vi "Get Server Stop Event.vi"(8 "error in (no error)":errorcluster, 11 "Base Server in":refnum<class "Server.lvclass">) -> (0 "error out":errorcluster, 3 "Server Stop Event":refnum<user-event>)   [LabVIEW 2024, in "Ramses Framework.lvlib" / "Server.lvclass"]
uses:
  Server.lvclass
  Server.lvclass/Server.ctl
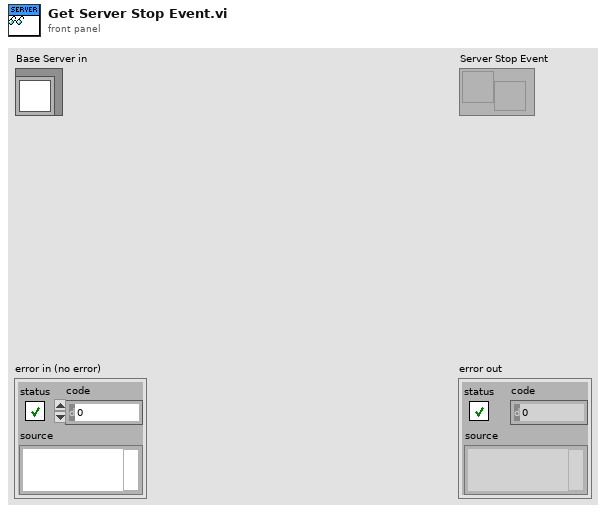
[diagram p1: front panel]
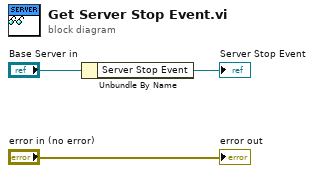
[diagram p0: block diagram]
diagram:
  n1 = Unbundle By Name("Base Server in") -> ("Server Stop Event"=→"Server Stop Event":refnum<user-event>)
  "error out" <- "error in (no error)"
